vi "MS Operation IOP Ctrl Local Cmd.vi"(6 "PID Cluster":T3={"L1 to L4 PID Cluster"={"L1 PID Gains"={"Kp"=0.005, "Kd"=0.5, "Ki"=0.0005}, "L2 PID Gains"={"Kp"=0.01, "Kd"=1.0, "Ki"=0.005}, "L3 PID Gains"={"Kp"=0.05, "Kd"=1.0, "Ki"=0.0005}, "L4 PID Gains"={"Kp"=0.1, "Kd"=0.1, "Ki"=0.0005}}, "Stage PID Cluster"={"Stage Z PID"={"Kp"=0.0005, "Kd"=0.001, "Ki"=0.0}, "Stage Y PID"={"Kp"=0.0003, "Kd"=0.01, "Ki"=0.0}, "Stage X PID"={"Kp"=0.0003, "Kd"=0.01, "Ki"=0.0}}, "OCT Z PID Gains"={"Kp"=0.0003, "Kd"=0.0001, "Ki"=0.01}}, 7 "Robot Command":dbl[](array[numeric])=[0.0, 0.0, 0.0, 0.0], 8 "error in":errorcluster, 9 "Offset Home 2 RCM":dbl[](array[numeric])=[0.0, 0.0, 0.0, 0.0], 10 "Prev Posit Cluster":T2={"Prev L1 to L4 Posit"=[-0.5319, -0.035669172703475985, -2.0566170657346783, 0.9099264705882353], "Prev Stage Posit"=[6.002553885707208, 5.996566124542428, 5.995469940427586], "Prev OCT Z Posit"=-0.0}, 11 "FPGA VI Reference In":refnum<k20>) -> (0 "error out":errorcluster, 2 "Last Posit Cluster":T1={"Last L1 to L4 Posit"=[0.0, 0.0, 0.0, 0.0], "Last Stage Posit"=[6.0, 6.0, 6.0], "Last OCT Z Posit"=0.0}, 3 "FPGA VI Reference Out":refnum<k20>)   [LabVIEW 2016]
uses:
  Global Variables.vi
  <vilib>/Platform/TimedLoop/XDataNode/wakeup.ctl
  <vilib>/Platform/TimedLoop/XDataNode/XDNodeRunTimeDep.lvlib
  <vilib>/Platform/TimedLoop/XDataNode/nitl_modes.ctl
  <vilib>/Platform/TimedLoop/XDataNode/timing_clust.ctl
  <vilib>/platform/TimedLoop/XDataNode/XDataNode.xnode
  <vilib>/rvi/interface/nirviReadWriteControl/nirviReadWriteControl.xnode
  Library/KevinLibraryAll/labview/KevLib01.lvlib
  FPGA Bitfiles/PhantomControlPI_FPGATarget_QuadCtr2_E2412E44.lvbitx
  IRISS_FPGA_IO.vi
  <vilib>/Utility/error.llb/Error Cluster From Error Code.vi
  <vilib>/rvi/errors/niLvFpgaAdjustHostInterfaceError.vi
  Library/KevinLibraryAll/labview2011/kevLib2011.lvlib
  <vilib>/Utility/file.llb/Write Delimited Spreadsheet (string).vi
  <vilib>/Utility/file.llb/Write Delimited Spreadsheet (DBL).vi
  NiFpgaLv.dll
panel:
  out "Period [ms]":i64=10
  out "Acc Ctrl Array":dbl[](array[numeric])
  out "Acc Button 4":bool
  out "Accurus Remote cmd":T4
  out "L1 to L4 Remote cmd":sgl[](array[numeric])
  # "L1"
  # "L2"
  # "L3"
  # "L4"
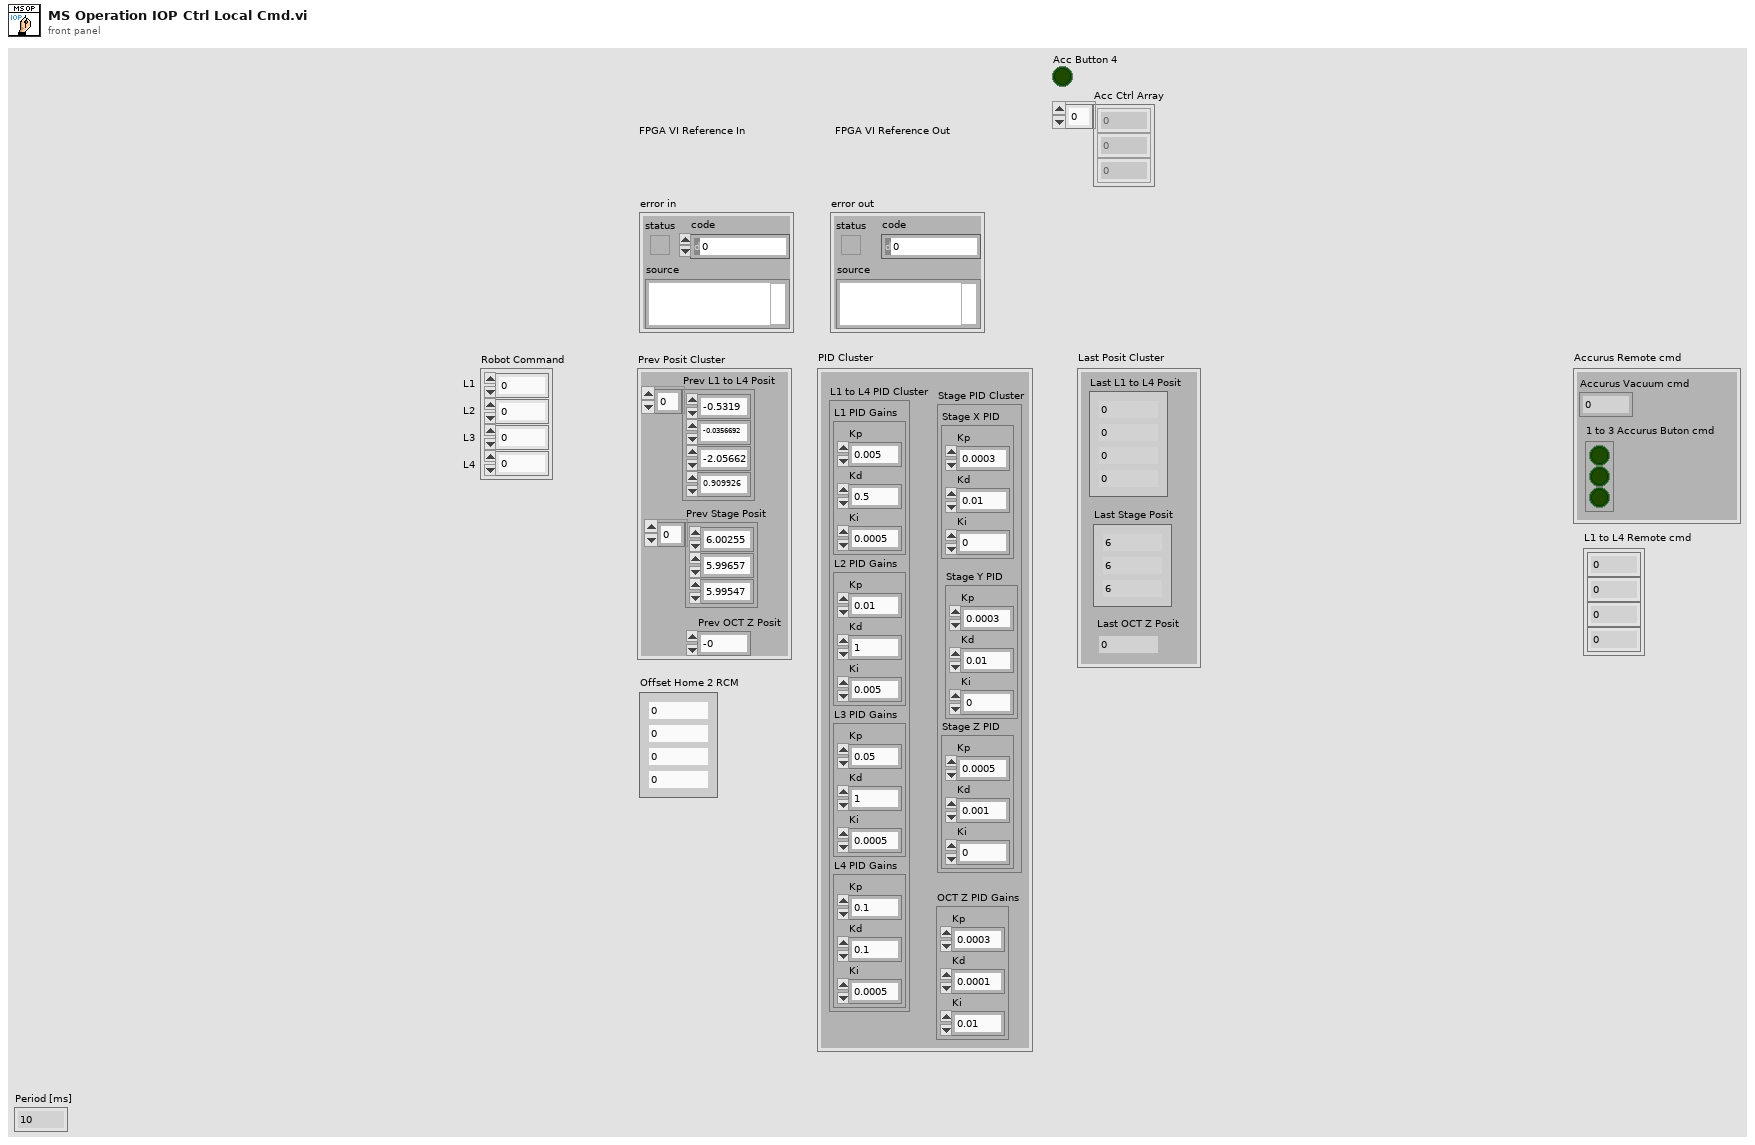
[diagram p1: front panel]
types:
  T1 = cluster{"Last L1 to L4 Posit":dbl[], "Last Stage Posit":dbl[], "Last OCT Z Posit":dbl}
  T2 = cluster{"Prev L1 to L4 Posit":dbl[], "Prev Stage Posit":dbl[], "Prev OCT Z Posit":dbl}
  T3 = cluster{"L1 to L4 PID Cluster":cluster{"L1 PID Gains":cluster{"Kp":dbl, "Kd":dbl, "Ki":dbl}, "L2 PID Gains":cluster{"Kp":dbl, "Kd":dbl, "Ki":dbl}, "L3 PID Gains":cluster{"Kp":dbl, "Kd":dbl, "Ki":dbl}, "L4 PID Gains":cluster{"Kp":dbl, "Kd":dbl, "Ki":dbl}}, "Stage PID Cluster":cluster{"Stage Z PID":cluster{"Kp":dbl, "Kd":dbl, "Ki":dbl}, "Stage Y PID":cluster{"Kp":dbl, "Kd":dbl, "Ki":dbl}, "Stage X PID":cluster{"Kp":dbl, "Kd":dbl, "Ki":dbl}}, "OCT Z PID Gains":cluster{"Kp":dbl, "Kd":dbl, "Ki":dbl}}
  T4 = cluster{"Accurus Vacuum cmd":sgl, "1 to 3 Accurus Buton cmd":bool[]}
  T5 = cluster{"Accurus button":bool[], "Accurus engaged?":bool, "Vacuum Force":i32, "Accurus Ch. A Vout":dbl, "Accurus Ch. B Vout":dbl, "Irrigation engaged?":bool}
  T6 = typedef "XDNodeRunTimeDep.lvlib/timing_clust.ctl" = cluster{"Expected End [f-1]":u64, "Actual End [f-1]":u64, "Finished Late? [f-1]":bool, "Expected End [i-1]":u64, "Actual End [i-1]":u64, "Finished Late? [i-1]":bool, "Expected Start [i]":u64, "Actual Start [i]":u64, "Expected Start [f]":u64, "Actual Start [f]":u64, "Source Name":string, "Structure Name":string, "Period":i64, "Deadline":i64, "Offset":i64, "Start":i64, "Priority":i32, "Timeout":i32, "Mode":T7, "Wakeup Reason":T8, "Error":errorcluster, "Source Type":string, "Secondary Source Type":string, "Global End Time":u64, "Global Start Time":u64, "Frame Duration":u64, "Iteration Duration":u64, "Assigned CPU":i32, "I/O Scan Engine Mode":u32}
  T7 = typedef "XDNodeRunTimeDep.lvlib/nitl_modes.ctl" = enum32{"No Change", "Process missed periods, maintain original phase", "Discard missed periods, maintain original phase", "Process missed periods, ignore original phase", "Discard missed periods, ignore original phase"}
  T8 = typedef "XDNodeRunTimeDep.lvlib/wakeup.ctl" = enum32{"Normal", "Aborted", "Asynchronous wakeup", "Timing source error", "Timed loop error", "Timeout"}
  T9 = cluster{"L1 PID Gains":cluster{"Kp":dbl, "Kd":dbl, "Ki":dbl}, "L2 PID Gains":cluster{"Kp":dbl, "Kd":dbl, "Ki":dbl}, "L3 PID Gains":cluster{"Kp":dbl, "Kd":dbl, "Ki":dbl}, "L4 PID Gains":cluster{"Kp":dbl, "Kd":dbl, "Ki":dbl}}
  T10 = cluster{"Stage Z PID":cluster{"Kp":dbl, "Kd":dbl, "Ki":dbl}, "Stage Y PID":cluster{"Kp":dbl, "Kd":dbl, "Ki":dbl}, "Stage X PID":cluster{"Kp":dbl, "Kd":dbl, "Ki":dbl}}
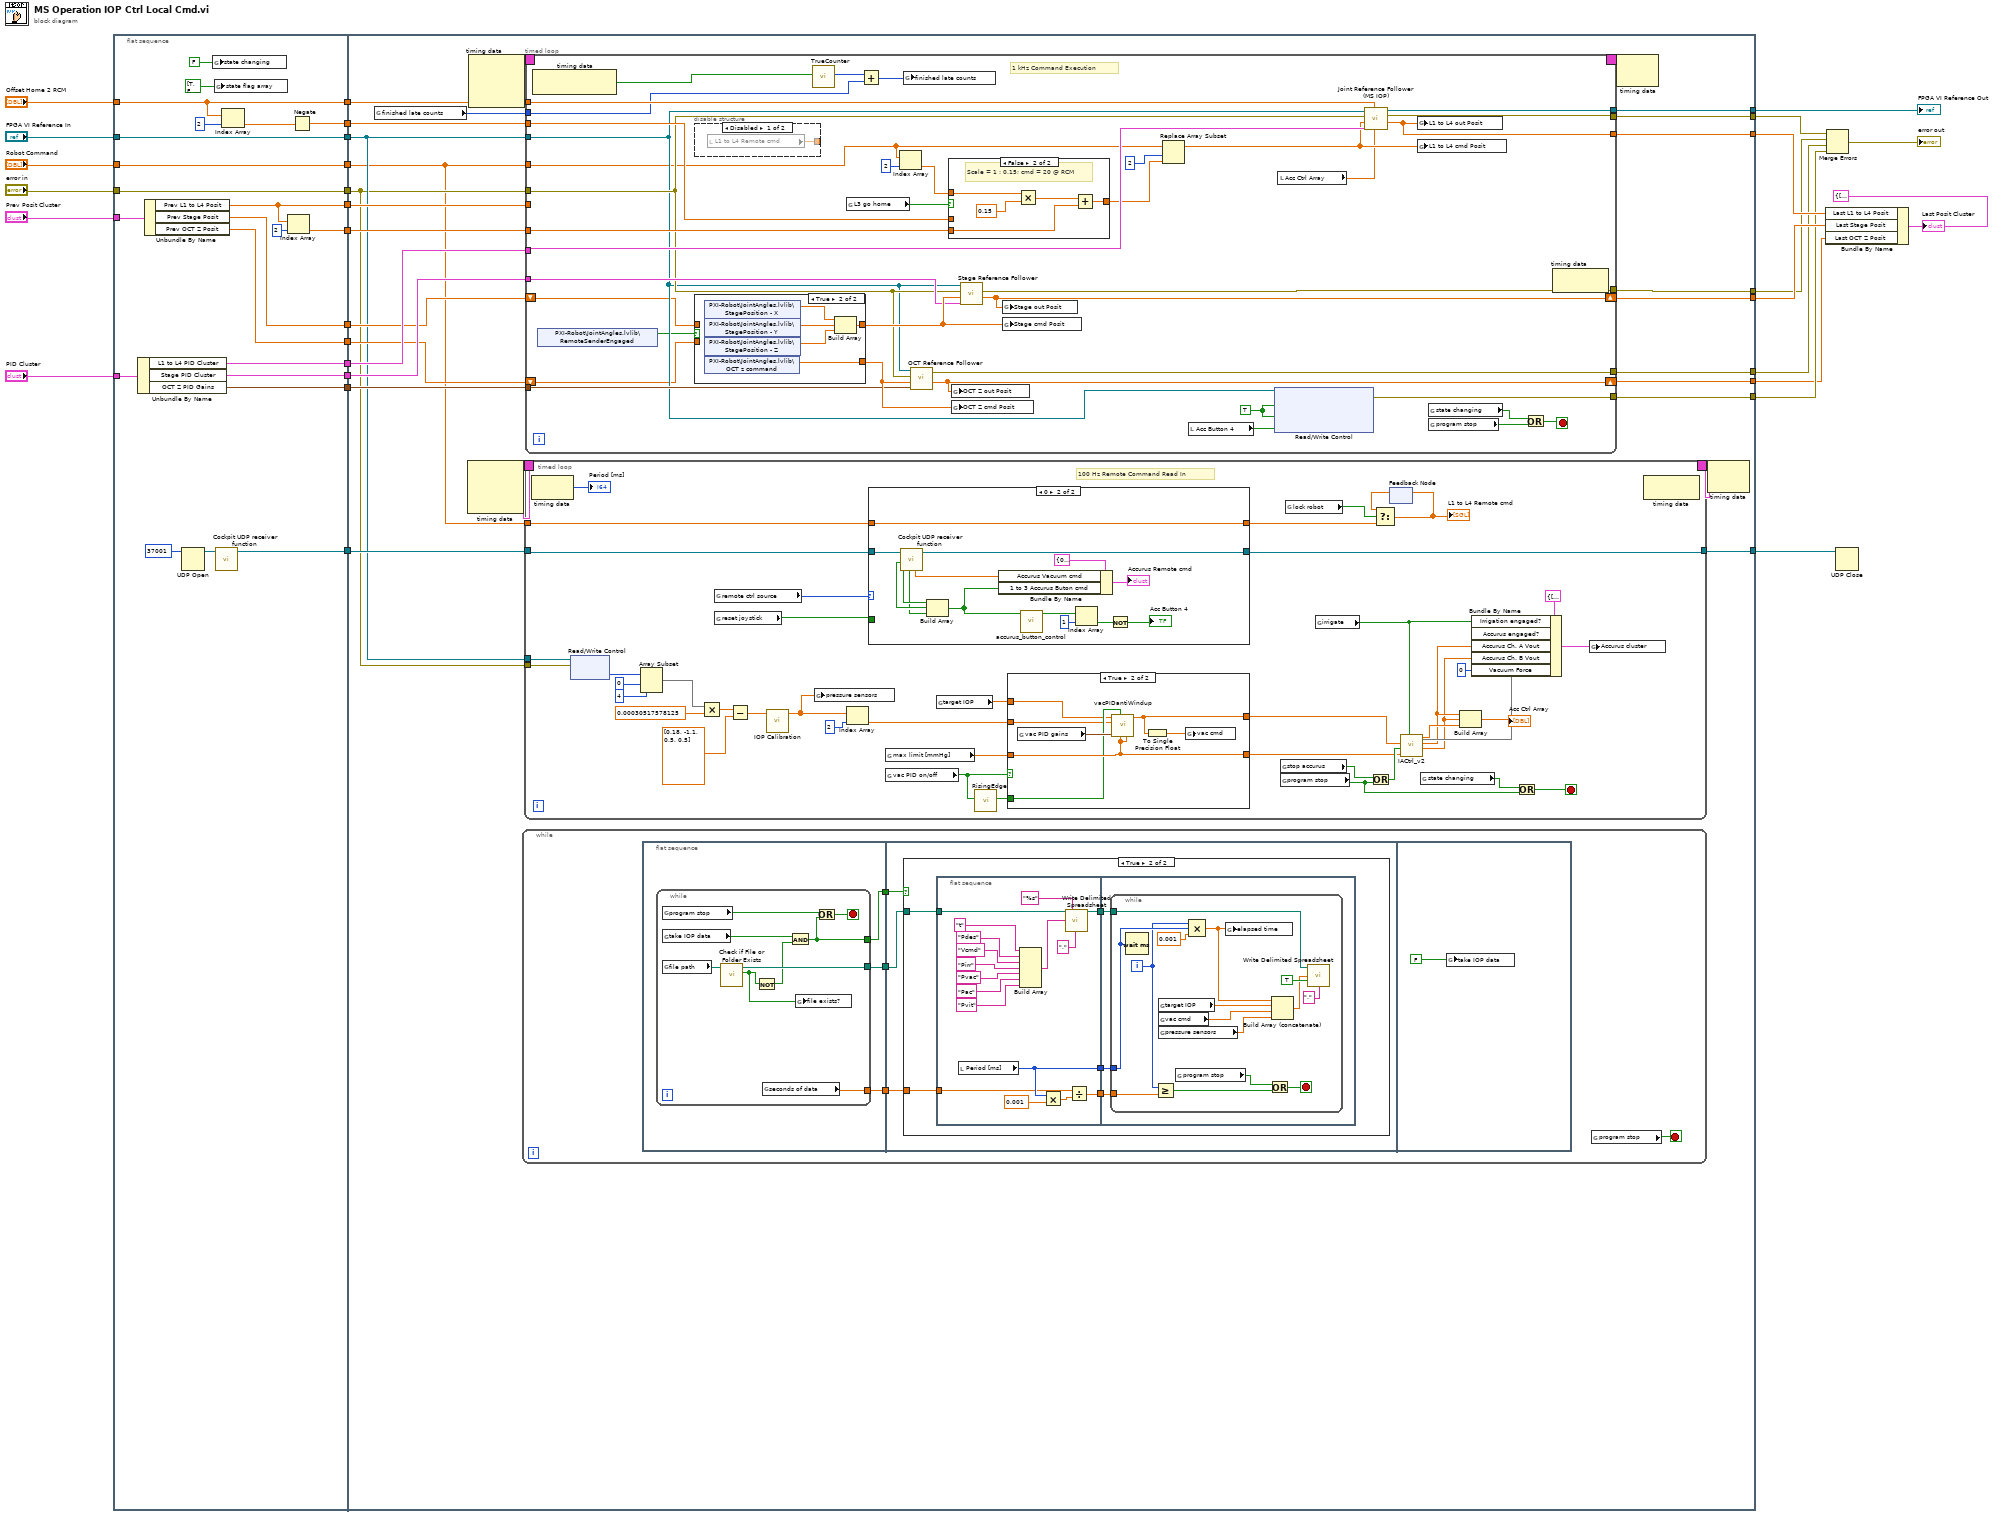
[diagram p0: block diagram]
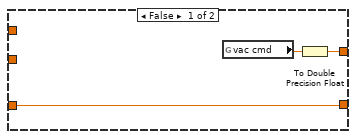
[diagram p3: hidden frame]
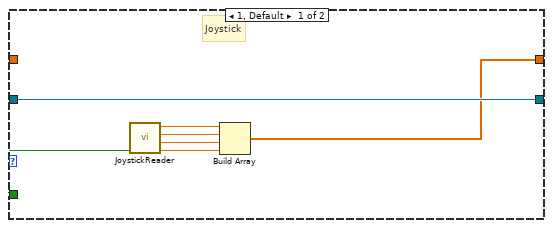
[diagram p4: hidden frame]
diagram:
  n1 = flat-sequence {
    tunnel: [w49] -> w31
    tunnel: [w48] -> w29
    tunnel: "FPGA VI Reference In" -> [w48]
    tunnel: [w47] -> w27
    tunnel: "error in" -> [w47]
    tunnel: [w40] -> w25
    tunnel: "Offset Home 2 RCM" -> [w40]
    tunnel: "Prev Posit Cluster" -> [w35]
    tunnel: [w45] -> w22
    tunnel: "PID Cluster" -> [w44]
    tunnel: [w43] -> w20
    tunnel: [w42] -> w19
    tunnel: [w38] -> w18
    tunnel: [w37] -> w6
    tunnel: [w36] -> w5
    tunnel: [w34] -> w4
    tunnel: [w33] -> w3
    tunnel: [w32] -> w2
    tunnel: "Robot Command" -> [w32]
    tunnel: w31 -> [w76]
    tunnel: [w75] -> w30
    tunnel: w29 -> [w56]
    tunnel: w27 -> [w55]
    tunnel: w25 -> [w74]
    tunnel: w22 -> [w73]
    tunnel: w20 -> [w72]
    tunnel: w19 -> [w71]
    tunnel: w18 -> [w70]
    tunnel: [w69] -> w8
    tunnel: [w68] -> w14
    tunnel: [w67] -> w15
    tunnel: [w57] -> w12
    tunnel: [w58] -> w11
    tunnel: [w66] -> w9
    tunnel: [w65] -> w10
    tunnel: [w59] -> w7
    tunnel: w6 -> [w64]
    tunnel: w5 -> [w63]
    tunnel: w4 -> [w61]
    tunnel: w3 -> [w60]
    tunnel: w2 -> [w54]
    frame #0 {
      n2 = Unbundle By Name(w44) -> ("L1 to L4 PID Cluster"=w43:T9, "Stage PID Cluster"=w37:T10, "OCT Z PID Gains"=w36:cluster{"Kp":dbl, "Kd":dbl, "Ki":dbl})
      n3 = Unbundle By Name(w35) -> ("Prev L1 to L4 Posit"=w45:dbl[], "Prev Stage Posit"=w34:dbl[], "Prev OCT Z Posit"=w33:dbl)
      n4 = UDP Open(11:u16 37001 ("port")) -> (port=w51:refnum<k16>)  [unwired: 4 in, 2 out]
      n5 = global write "Global Variables.vi" "state changing"(FALSE ("state changing")) -> ()
      n6 = global write "Global Variables.vi" "state flag array"(bool[] [TRUE, FALSE, FALSE, FALSE, FALSE, FALSE, FALSE, FALSE, FALSE] ("state flag array")) -> ()
      n7 = call "Cockpit UDP receiver function.vi"("UDP connection ID"=w51) -> ("UDP connection ID out"=w49:refnum<k16>)  [unwired: 1 in, 9 out]
      n8 = Index Array(array=w40, index=2) -> (element=w39:dbl)
      n9 = Index Array(array=w45, index=2) -> (element=w42:dbl)
      n10 = Negate(x=w39) -> (-x=w38:dbl)
    }
    frame #1 {
      n11 = global read "Global Variables.vi" "finished late counts"() -> (w62:u16)
      n12 = node-c288() -> (w78:T6)  [unwired: 3 in]
      n13 = node-c288() -> (w80:T6)  [unwired: 3 in]
      n14 = while {
        stop <- w81 stop-if-true
        n15 = flat-sequence {
          tunnel: [w85] -> w84
          tunnel: [w87] -> w83
          tunnel: [w86] -> w82
          tunnel: w84 -> [w99]
          tunnel: w83 -> [w98]
          tunnel: w82 -> [w97]
          frame #0 {
            n16 = while {
              tunnel: [w95] -> w87
              tunnel: [w88] -> w86
              tunnel: [w93] -> w85
              stop <- w96 stop-if-true
              n17 = global read "Global Variables.vi" "program stop"() -> (w92:bool)
              n18 = global read "Global Variables.vi" "take IOP data"() -> (w91:bool)
              n19 = global read "Global Variables.vi" "file path"() -> (w90:path)
              n20 = call <vilib>:"Check if File or Folder Exists.vi"("path"=w90) -> ("file or folder exists?"=w89:bool, "dup path"=w95:path)  [unwired: 8 in, 1 out]
              n21 = Not(x=w89) -> (.not. x?=w94:bool)
              n22 = global read "Global Variables.vi" "seconds of data"() -> (w88:sgl)
              n23 = And(x=w91, y=w94) -> (x .and. y?=w93:bool)
              n24 = global write "Global Variables.vi" "file exists?"(w89) -> ()
              n25 = Or(x=w92, y=w93) -> (x .or. y?=w96:bool)
            }
          }
          frame #1 {
            n26 = case shown="True" w99 {
              tunnel: w98 -> [_ w104]
              tunnel: w97 -> [_ w101]
              frame False {
              }
              frame True {
                n27 = flat-sequence {
                  tunnel: w104 -> [w110]
                  tunnel: [w108] -> w103
                  tunnel: [w119] -> w102
                  tunnel: w101 -> [w118]
                  tunnel: [w116] -> w100
                  tunnel: w103 -> [w124]
                  tunnel: w102 -> [w123]
                  tunnel: w100 -> [w122]
                  frame #0 {
                    n28 = local read "Period [ms]"() -> (w119:i64)
                    n29 = Build Array("t" ("delimiter (\\t)"), "Pdes" ("delimiter (\\t)"), "Vcmd" ("delimiter (\\t)"), "Pirr" ("delimiter (\\t)"), "Pvac" ("delimiter (\\t)"), "Pac" ("delimiter (\\t)"), "Pvit" ("delimiter (\\t)")) -> (w107:string[])
                    n30 = Multiply(x=w119, y=0.001) -> (x*y=w117:dbl)
                    n31 = call-poly <vilib>:"Write Delimited Spreadsheet.vi"("file path (dialog if empty)"=w110, "format (%s)"="%s", "1D data"=w107, "delimiter (\\t)"="," ("delimiter (\\t)")) -> ("new file path (Not A Path if cancelled)"=w108:path)  [unwired: 10 in, 1 out]
                    n32 = Divide(x=w118, y=w117) -> (x/y=w116:dbl)
                  }
                  frame #1 {
                    n33 = while {
                      tunnel: w124 -> [w133]
                      tunnel: w123 -> [w137]
                      tunnel: w122 -> [w135]
                      i -> [w136]
                      stop <- w139 stop-if-true
                      n34 = Wait (ms)(milliseconds to wait=w137) -> ()  [unwired: 1 out]
                      n35 = Greater Or Equal?(x=w136, y=w135) -> (x >= y?=w134:bool)
                      n36 = global read "Global Variables.vi" "target IOP"() -> (w125:sgl)
                      n37 = global read "Global Variables.vi" "vac cmd"() -> (w128:sgl)
                      n38 = global read "Global Variables.vi" "pressure sensors"() -> (w127:sgl[])
                      n39 = global read "Global Variables.vi" "program stop"() -> (w129:bool)
                      n40 = Compound Arithmetic op=MULTIPLY(w136, w137, 0.001 ("y")) -> (w126:dbl)
                      n41 = global write "Global Variables.vi" "elapsed time"(w126) -> ()
                      n42 = Or(x=w129, y=w134) -> (x .or. y?=w139:bool)
                      n43 = Build Array (concatenate)(w126, w125, w128, w127) -> (w131:dbl[])
                      n44 = call-poly <vilib>:"Write Delimited Spreadsheet.vi"("file path (dialog if empty)"=w133, "1D data"=w131, "append to file? (new file:F)"=TRUE, "delimiter (\\t)"="," ("delimiter (\\t)")) -> ()  [unwired: 10 in, 2 out]
                    }
                  }
                }
              }
            }
          }
          frame #2 {
            n45 = global write "Global Variables.vi" "take IOP data"(FALSE) -> ()
          }
        }
        n46 = global read "Global Variables.vi" "program stop"() -> (w81:bool)
      }
      n47 = timed-loop {
        timing: w78 -> [_]
        timing-out: [_] -> w77
        tunnel: w76 -> [w181]
        tunnel: [w180] -> w75
        tunnel: w56 -> [w172]
        tunnel: w55 -> [w171]
        tunnel: w54 -> [w141]
        stop <- w183 stop-if-true
        # "100 Hz Remote Command Read In"
        n48 = node-c288() -> (→"Period [ms]":i64)  [unwired: 1 in]
        n49 = xnode "Read/Write Control"("FPGA VI Reference In"=w172, "error in"=w171) -> ("AI"=w163:i16[])  [unwired: 2 out]
        n50 = Array Subset(array=w163, index=0, length=4) -> (w168:i16[])
        n51 = Multiply(x=w168, y=0.00030517578125) -> (x*y=w169:dbl[])
        n52 = global read "Global Variables.vi" "remote ctrl source"() -> (w179:u16)
        n53 = global read "Global Variables.vi" "reset joystick"() -> (w178:bool)
        n54 = Subtract(x=w169, y=dbl[] [0.18, -1.1, 0.5, 0.5]) -> (x-y=w164:dbl[])
        n55 = call "IOP Calibration.vi"("IOP Input [V]"=w164) -> ("IOP Output [mmHg]"=w153:dbl[])  [unwired: 10 in]
        n56 = global write "Global Variables.vi" "pressure sensors"(w153) -> ()
        n57 = Index Array(array=w153, index=2) -> (element=w161:dbl)
        n58 = case shown="0" w179 {
          tunnel: [w199 w214] -> w180
          tunnel: w181 -> [w199 w208]
          tunnel: w178 -> [w200 _]
          tunnel: [w194 w201] -> w174
          tunnel: w141 -> [_ w201]
          frame 1, Default {
            # "Joystick"
            n59 = call "JoystickReader.vi"("Reset"=w200) -> ("L4 [deg]"=w195:sgl, "L3 [0~100]"=w196:sgl, "L2 [deg]"=w197:sgl, "L1 [deg]"=w198:sgl)  [unwired: 7 in]
            n60 = Build Array(w198, w197, w196, w195) -> (w194:sgl[])
          }
          frame 0 {
            n61 = call "Cockpit UDP receiver function.vi"("UDP connection ID"=w208) -> ("UDP connection ID out"=w214:refnum<k16>, "down_pedal"=w207:sgl, "right_pedal"=w209:bool, "left_pedal"=w211:bool, "up_pedal"=w210:bool)  [unwired: 1 in, 5 out]
            n62 = Build Array(w211, w210, w209) -> (w202:bool[])
            n63 = Bundle By Name(cluster=T4 {"Accurus Vacuum cmd"=0.0, "1 to 3 Accurus Buton cmd"=[FALSE, FALSE, FALSE]} ("Accurus Cockpit cmd 2"), "Accurus Vacuum cmd"=w207, "1 to 3 Accurus Buton cmd"=w202) -> (→"Accurus Remote cmd":T4)
            n64 = call "accurus_button_control.vi"("Array in"=w202) -> ("Array out"=w205:bool[])  [unwired: 10 in]
            n65 = Index Array(array=w205, index=1) -> (element=w204:bool)
            n66 = Not(x=w204) -> (.not. x?=→"Acc Button 4":bool)
          }
        }
        n67 = global read "Global Variables.vi" "max limit [mmHg]"() -> (w155:dbl)
        n68 = global read "Global Variables.vi" "vac PID on/off"() -> (w144:bool)
        n69 = global read "Global Variables.vi" "target IOP"() -> (w160:sgl)
        n70 = call "RisingEdge.vi"("Signal In"=w144) -> ("Rising Edge"=w143:bool)  [unwired: 10 in]
        n71 = case shown="True" w144 {
          tunnel: w161 -> [_ w187]
          tunnel: w160 -> [_ w188]
          tunnel: [w184 w192] -> w142
          tunnel: w155 -> [w186 w190]
          tunnel: [w186 w190] -> w154
          tunnel: w143 -> [_ w189]
          frame False {
            n72 = global read "Global Variables.vi" "vac cmd"() -> (w185:sgl)
            n73 = To Double Precision Float(number=w185) -> (double precision float=w184:dbl)
          }
          frame True {
            n74 = global read "Global Variables.vi" "vac PID gains"() -> (w191:cluster{"Kp":dbl, "Kd":dbl, "Ki":dbl, "Ts":dbl})
            n75 = call "vacPIDantiWindup.vi"("Saturation U"=w190, "Saturation M"=w190, "Reset"=w189, "PID Gains"=w191, "Feedback"=w187, "Reference"=w188) -> ("Control"=w192:dbl)  [unwired: 5 in]
            n76 = To Single Precision Float(number=w192) -> (single precision float=w193:sgl)
            n77 = global write "Global Variables.vi" "vac cmd"(w193) -> ()
          }
        }
        n78 = global read "Global Variables.vi" "stop accurus"() -> (w173:bool)
        n79 = global read "Global Variables.vi" "program stop"() -> (w156:bool)
        n80 = global read "Global Variables.vi" "lock robot"() -> (w177:bool)
        n81 = global read "Global Variables.vi" "irrigate"() -> (w149:bool)
        n82 = Or(x=w173, y=w156) -> (x .or. y?=w157:bool)
        n83 = feedback #1() -> (w176:dbl[])  [unwired: 1 in]
        n84 = Select(t=w176, s=w177, f=w174) -> (s? t:f=w175:dbl[])
        "L1 to L4 Remote cmd" <- w175
        n85 = feedback-in #1(w175) -> ()
        n86 = call "IACtrl_v2.vi"("Irrigate?"=w149, "Max Limit [mmHg]"=w154, "E-Stop Vacuum"=w157, "Vacuum Force [mmHg]"=w142) -> ("Accurus ChB Vout"=w147:dbl, "Accurus ChA Vout"=w148:dbl, "Accurus Engaged Vout"=w159:dbl, 5:w150)  [unwired: 3 in, 1 out]
        n87 = global read "Global Variables.vi" "state changing"() -> (w182:bool)
        n88 = Build Array(w148, w147, w159) -> (→"Acc Ctrl Array":dbl[])
        n89 = Bundle By Name(cluster=T5 {"Accurus button"=[FALSE, FALSE, FALSE], "Accurus engaged?"=FALSE, "Vacuum Force"=0, "Accurus Ch. A Vout"=0.0, "Accurus Ch. B Vout"=0.0, "Irrigation engaged?"=FALSE} ("Accurus Output Cluster"), "Irrigation engaged?"=w149, "Accurus engaged?"=w150, "Accurus Ch. A Vout"=w148, "Accurus Ch. B Vout"=w147, "Vacuum Force"=0) -> (w151:T5)
        n90 = Or(x=w182, y=w156) -> (x .or. y?=w183:bool)
        n91 = global write "Global Variables.vi" "Accurus cluster"(w151) -> ()
        n92 = node-c288() -> ()  [unwired: 1 in, 1 out]
      }
      n93 = timed-loop {
        timing: w80 -> [_]
        timing-out: [_] -> w79
        tunnel: w56 -> [w230]
        tunnel: w55 -> [w231]
        tunnel: w74 -> [w252]
        tunnel: w73 -> [_]
        tunnel: w72 -> [w249]
        tunnel: w71 -> [w248]
        tunnel: w70 -> [w245]
        tunnel: [w244] -> w69
        tunnel: [w243] -> w68
        tunnel: [w242] -> w67
        tunnel: [w241] -> w66
        tunnel: [w240] -> w65
        tunnel: w64 -> [w237]
        tunnel: w63 -> [w236]
        tunnel: w62 -> [w232]
        shift-right: [w226] -> w58
        shift-left: w61 -> [w229]
        shift-right: [w227] -> w59
        shift-left: w60 -> [w228]
        tunnel: [w224] -> w57
        tunnel: w54 -> [w220]
        stop <- w257 stop-if-true
        w239 = TRUE ("Conn0/DIO15 Button 4")
        # "1 kHz Command Execution"
        n94 = node-c288() -> (w235:bool)  [unwired: 1 in]
        n95 = shared-variable "PXI-Robot\\JointAngles.lvlib\\RemoteSenderEngaged"() -> (w225:bool)  [unwired: 1 in, 1 out]
        n96 = case shown="True" w225 {
          tunnel: [w260 w265] -> w251
          tunnel: [w259 w261] -> w250
          tunnel: w229 -> [w260 _]
          tunnel: w228 -> [w259 _]
          frame False {
          }
          frame True {
            n97 = shared-variable "PXI-Robot\\JointAngles.lvlib\\StagePosition - X"() -> (w262:dbl)  [unwired: 1 in, 1 out]
            n98 = shared-variable "PXI-Robot\\JointAngles.lvlib\\StagePosition - Y"() -> (w263:dbl)  [unwired: 1 in, 1 out]
            n99 = shared-variable "PXI-Robot\\JointAngles.lvlib\\StagePosition - Z"() -> (w264:dbl)  [unwired: 1 in, 1 out]
            n100 = shared-variable "PXI-Robot\\JointAngles.lvlib\\OCT z command"() -> (w261:dbl)  [unwired: 1 in, 1 out]
            n101 = Build Array(w262, w263, w264) -> (w265:dbl[])
          }
        }
        n102 = disable-structure shown="Disabled" {
          disable-tunnel: [w258 _] -> _
          frame Disabled {
            n103 = local read "L1 to L4 Remote cmd"() -> (w258:sgl[])
          }
          frame Enabled {
          }
        }
        n104 = call "TrueCounter.vi"("True?"=w235) -> ("True Count"=w233:u16)  [unwired: 10 in]
        n105 = global read "Global Variables.vi" "L3 go home"() -> (w255:bool)
        n106 = Add(x=w233, y=w232) -> (x+y=w234:u16)
        n107 = Index Array(array=w220, index=2) -> (element=w253:dbl)
        n108 = global write "Global Variables.vi" "finished late counts"(w234) -> ()
        n109 = call "OCT Reference Follower.vi"("OCT Z PID Gains"=w236, "OCT  Z cmd Posit [mm]"=w250, "error in"=w231, "FPGA VI Reference In"=w230) -> ("OCT  Z out Posit [mm]"=w227:dbl, "error out"=w241:errorcluster)  [unwired: 5 in, 1 out]
        n110 = case shown="False" w255 {
          tunnel: [w266 w271] -> w246
          tunnel: w253 -> [_ w268]
          tunnel: w248 -> [_ w267]
          tunnel: w245 -> [w266 _]
          frame True {
            # "Go Home"
          }
          frame False {
            # "Scale = 1 : 0.15; cmd = 20 @ RCM"
            n111 = Multiply(x=w268, y=0.15) -> (x*y=w270:dbl)
            n112 = Add(x=w270, y=w267) -> (x+y=w271:dbl)
          }
        }
        n113 = global write "Global Variables.vi" "OCT Z out Posit"(w227) -> ()
        n114 = global write "Global Variables.vi" "OCT Z cmd Posit"(w250) -> ()
        n115 = call "Stage Reference Follower.vi"("Stage PID Cluster"=w237, "Stage cmd Posit [mm]"=w251, "error in"=w231, "FPGA VI Reference In"=w230) -> ("Stage out Posit [mm]"=w226:dbl[], "error out"=w240:errorcluster)  [unwired: 5 in, 1 out]
        n116 = global write "Global Variables.vi" "Stage out Posit"(w226) -> ()
        n117 = global write "Global Variables.vi" "Stage cmd Posit"(w251) -> ()
        n118 = Replace Array Subset(array=w220, new element=w246, index=2) -> (w223:dbl[])
        n119 = local read "Acc Button 4"() -> (w221:bool)
        n120 = xnode "Read/Write Control"("FPGA VI Reference In"=w230, "Conn0/DIO12 Button 1"=w239, "Conn0/DIO13 Button 2"=w239, "Conn0/DIO15 Button 4"=w221) -> ("error out"=w244:errorcluster)  [unwired: 1 in, 1 out]
        n121 = local read "Acc Ctrl Array"() -> (w222:dbl[])
        n122 = call "Joint Reference Follower (MS IOP).vi"("Acc Ctrl Array"=w222, "Offset Home2RCM [deg/mm]"=w252, "PID Ctrl Cluster"=w249, "Ref Array [deg/mm]"=w223, "error in"=w231, "FPGA VI Reference In"=w230) -> ("Output Posit Array [deg/mm]"=w224:dbl[], "error out"=w243:errorcluster, "FPGA VI Reference Out"=w242:refnum<k20>)  [unwired: 3 in]
        n123 = global write "Global Variables.vi" "L1 to L4 out Posit"(w224) -> ()
        n124 = global write "Global Variables.vi" "L1 to L4 cmd Posit"(w223) -> ()
        n125 = global read "Global Variables.vi" "state changing"() -> (w256:bool)
        n126 = global read "Global Variables.vi" "program stop"() -> (w238:bool)
        n127 = Or(x=w256, y=w238) -> (x .or. y?=w257:bool)
        n128 = node-c288() -> ()  [unwired: 1 in, 1 out]
      }
      n129 = node-c288(w79) -> ()  [unwired: 1 out]
      n130 = node-c288(w77) -> ()  [unwired: 1 out]
    }
  }
  n131 = Bundle By Name(cluster=T1 {"Last L1 to L4 Posit"=[-0.5607, -0.038216970753724266, -2.0806193533568895, 1.1787683823529411], "Last Stage Posit"=[6.002553885707208, 5.996566124542428, 5.995469940427586], "Last OCT Z Posit"=-0.0} ("Last Posit Cluster 2"), "Last L1 to L4 Posit"=w12, "Last Stage Posit"=w11, "Last OCT Z Posit"=w7) -> (→"Last Posit Cluster":T1)
  n132 = Merge Errors(w14, w10, w9, w8) -> (→"error out":errorcluster)
  n133 = UDP Close(connection ID=w30) -> ()  [unwired: 1 in, 2 out]
  "FPGA VI Reference Out" <- w15
